vi "Set IConfiguration.vi"(10 "IConfiguration":refnum<class "IConfiguration.lvclass">, 11 "IMAQdx Base Configure Strategy in":refnum<class "IMAQdx Base Configure Strategy.lvclass">) -> (3 "IMAQdx Base Configure Strategy out":refnum<class "IMAQdx Base Configure Strategy.lvclass">)   [LabVIEW 2024, in "IMAQdx Base Configure Strategy.lvclass"]
uses:
  IMAQdx Base Configure Strategy.lvclass
  Source/Interfaces/IConfiguration/IConfiguration.lvclass
  IMAQdx Base Configure Strategy.lvclass/IMAQdx Base Configure Strategy.ctl
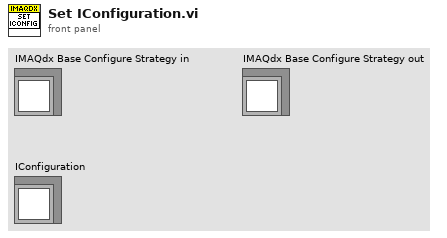
[diagram p1: front panel]
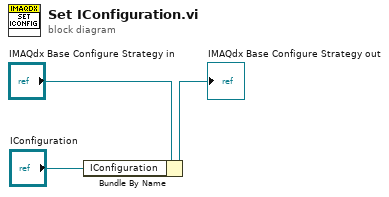
[diagram p0: block diagram]
diagram:
  n1 = Bundle By Name(cluster="IMAQdx Base Configure Strategy in", "IConfiguration"="IConfiguration") -> (→"IMAQdx Base Configure Strategy out":refnum<class "IMAQdx Base Configure Strategy.lvclass">)
